vi "WPI_DigitalOutputPWMAllocator.vi"(7 "Operation":T3, 8 "error in (no error)":errorcluster, 9 "DIO Channel":T1=enum."Invalid", 11 "PWM To Release":T2=enum."Invalid") -> (0 "error out":errorcluster, 1 "DIO Channel Out":T1=enum."DIO 1", 2 "Allocated":bool, 3 "PWM Allocated":T2=enum."DO PWM 1")   [LabVIEW 2017]
doc: "This software is licensed. Open the labview\\readme\\WPI Robotics Library Open Source License.txt file for more information."
uses:
  <vilib>/Rock Robotics/WPI/DigitalModule/WPI_DigitalModuleDIOCacheOp.ctl
  <vilib>/Rock Robotics/WPI/DigitalOutput/WPI_DigitalOutputPWMRef.ctl
  <vilib>/Rock Robotics/SystemInterfaces/DIO/FPGA_DIOChannel.ctl
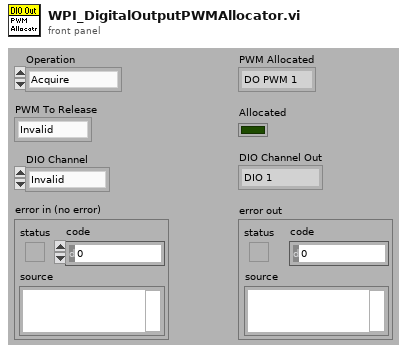
[diagram p1: front panel]
types:
  T1 = typedef "FPGA_DIOChannel.ctl" = enum8{"DIO 0", "DIO 1", "DIO 2", "DIO 3", "DIO 4", "DIO 5", "DIO 6", "DIO 7", "DIO 8", "DIO 9", "DIO MXP 0", "DIO MXP 1", "DIO MXP 2", "DIO MXP 3", "DIO MXP 4", "DIO MXP 5", "DIO MXP 6", "DIO MXP 7", "DIO MXP 8", "DIO MXP 9", "DIO MXP 10", "DIO MXP 11", "DIO MXP 12", "DIO MXP 13", "DIO MXP 14", "DIO MXP 15", "SPI Port CS1", "SPI Port CS2", "SPI Port CS3", "SPI Port MISO", "SPI Port MOSI", "Invalid"}
  T2 = typedef "WPI_DigitalOutputPWMRef.ctl" = enum16{"DO PWM 0", "DO PWM 1", "DO PWM 2", "DO PWM 3", "DO PWM 4", "DO PWM 5", "Invalid"}
  T3 = typedef "WPI_DigitalModuleDIOCacheOp.ctl" = enum16{"Acquire", "Release", "Status"}
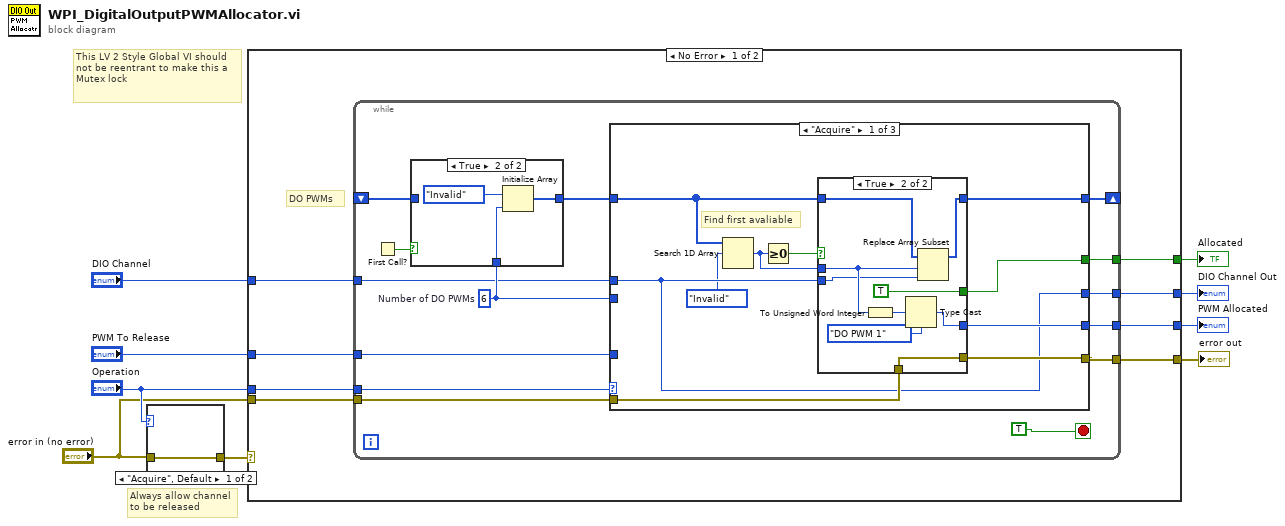
[diagram p0: block diagram]
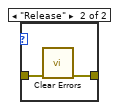
[diagram p2: hidden frame]
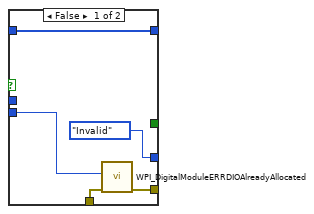
[diagram p3: hidden frame]
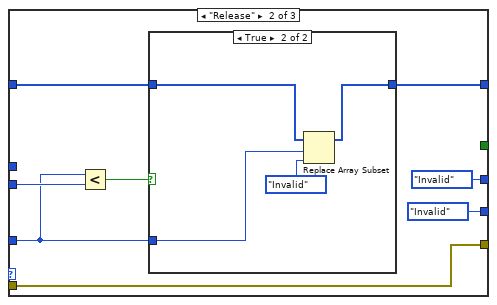
[diagram p4: hidden frame]
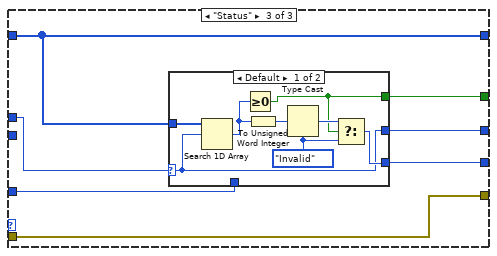
[diagram p6: hidden frame]
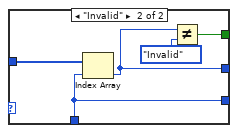
[diagram p7: hidden frame]
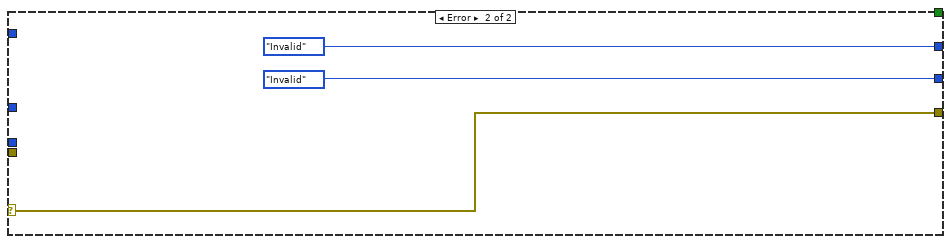
[diagram p9: hidden frame]
diagram:
  # "This LV 2 Style Global VI should not be reentrant to make this a Mutex lock"
  # "Always allow channel to be released"
  n1 = case shown="\"Acquire\", Default" "Operation" {
    tunnel: "error in (no error)" -> [w10 w12]
    tunnel: [w10 w11] -> w7
    frame "Acquire", Default {
    }
    frame "Release" {
      n2 = call <vilib>:"Clear Errors.vi"("error in (no error)"=w12) -> ("error out"=w11:errorcluster)  [unwired: 1 in, 5 out]
    }
  }
  n3 = case shown="No Error" w7 {
    selector: w7 -> [_ w98]
    tunnel: "Operation" -> [w20 _]
    tunnel: [w19 w98] -> w5
    tunnel: [w18 _] -> w9
    tunnel: [w17 WPI_DigitalOutputPWMRef."Invalid" ("DIOChannel Allocated")] -> w4
    tunnel: "error in (no error)" -> [w16 _]
    tunnel: "PWM To Release" -> [w15 _]
    tunnel: [w14 FPGA_DIOChannel."Invalid" ("DIO Channel")] -> w2
    tunnel: "DIO Channel" -> [w13 _]
    frame No Error {
      # "DO PWMs"
      n4 = while {
        shift-right: [w31] -> _
        shift-left: _ -> [w33]
        tunnel: w20 -> [w32]
        tunnel: [w30] -> w19
        tunnel: [w29] -> w18
        tunnel: [w27] -> w17
        tunnel: w16 -> [w25]
        tunnel: w15 -> [w24]
        tunnel: [w22] -> w14
        tunnel: w13 -> [w21]
        stop <- TRUE stop-if-true
        w23 = 6  # Number of DO PWMs
        n5 = First Call?() -> (First Call?: T/F=w34:bool)
        n6 = case shown="True" w34 {
          tunnel: w33 -> [w92 _]
          tunnel: [w92 w95] -> w28
          tunnel: w23 -> [_ w94]
          frame False {
          }
          frame True {
            n7 = Initialize Array(FPGA_DIOChannel."Invalid" ("DIO Channel"), w94) -> (w95:T1[])
          }
        }
        n8 = case shown="\"Acquire\"" w32 {
          tunnel: w28 -> [w41 w66 w77]
          tunnel: [w44 w65 w77] -> w31
          tunnel: [w43 w63 w78] -> w30
          tunnel: [w42 _ w76] -> w29
          tunnel: [w40 WPI_DigitalOutputPWMRef."Invalid" ("DIOChannel Allocated") w72] -> w27
          tunnel: w25 -> [w39 w63 w78]
          tunnel: w24 -> [_ w60 w73]
          tunnel: w23 -> [_ w62 _]
          tunnel: [w38 FPGA_DIOChannel."Invalid" ("DIO Channel") w75] -> w22
          tunnel: w21 -> [w38 _ w74]
          frame "Acquire" {
            # "Find first avaliable"
            n9 = Search 1D Array(1D array=w41, element=FPGA_DIOChannel."Invalid" ("DIO Channel")) -> (index of element=w37:i32)  [unwired: 1 out]
            n10 = Greater Or Equal To 0?(x=w37) -> (x >= 0?=w36:bool)
            n11 = case shown="True" w36 {
              tunnel: [_ TRUE ("new element/subarray")] -> w42
              tunnel: w41 -> [w49 w57]
              tunnel: [w49 w56] -> w44
              tunnel: w37 -> [_ w54]
              tunnel: [WPI_DigitalOutputPWMRef."Invalid" ("PWM Allocated") w52] -> w40
              tunnel: [w47 w51] -> w43
              tunnel: w39 -> [w46 w51]
              tunnel: w38 -> [w45 w50]
              frame False {
                n12 = call <vilib>:"WPI_DigitalModuleERRDIOAlreadyAllocated.vi"("error in (no error)"=w46, "DIOChannel"=w45) -> ("error out"=w47:errorcluster)  [unwired: 9 in]
              }
              frame True {
                n13 = To Unsigned Word Integer(number=w54) -> (unsigned 16bit integer=w55:u16)
                n14 = Type Cast(type=WPI_DigitalOutputPWMRef."DO PWM 1" ("PWM Allocated"), x=w55) -> (*(type *) &x=w52:T2)
                n15 = Replace Array Subset(array=w57, new element=w50, index=w54) -> (w56:T1[])
              }
            }
          }
          frame "Release" {
            n16 = Less?(x=w60, y=w62) -> (x < y?=w61:bool)
            n17 = case shown="True" w61 {
              tunnel: w66 -> [w67 w71]
              tunnel: w60 -> [_ w70]
              tunnel: [w67 w69] -> w65
              frame False {
              }
              frame True {
                n18 = Replace Array Subset(array=w71, new element=FPGA_DIOChannel."Invalid" ("DIO Channel"), index=w70) -> (w69:T1[])
              }
            }
          }
          frame "Status" {
            n19 = case shown="Default" w74 {
              selector: w74 -> [w80 _]
              tunnel: w77 -> [w86 w91]
              tunnel: [w83 w89] -> w76
              tunnel: [w80 w88] -> w75
              tunnel: w73 -> [_ w87]
              tunnel: [w81 w87] -> w72
              frame Default {
                w82 = WPI_DigitalOutputPWMRef."Invalid" ("PWM To Release")
                n20 = Search 1D Array(1D array=w86, element=w80) -> (index of element=w85:i32)  [unwired: 1 out]
                n21 = Greater Or Equal To 0?(x=w85) -> (x >= 0?=w83:bool)
                n22 = To Unsigned Word Integer(number=w85) -> (unsigned 16bit integer=w79:u16)
                n23 = Type Cast(type=w82, x=w79) -> (*(type *) &x=w84:T2)
                n24 = Select(t=w84, s=w83, f=w82) -> (s? t:f=w81:T2)
              }
              frame "Invalid" {
                n25 = Index Array(array=w91, index=w87) -> (element=w88:T1)
                n26 = Not Equal?(x=w88, y=FPGA_DIOChannel."Invalid" ("DIO Channel")) -> (x != y?=w89:bool)
              }
            }
          }
        }
      }
    }
    frame Error {
    }
  }
  "Allocated" <- w9
  "error out" <- w5
  "PWM Allocated" <- w4
  "DIO Channel Out" <- w2
